vi "GlobalSettings.vi"() -> ()   [LabVIEW 2015]
panel:
  out "Disable Write":bool
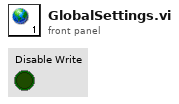
[diagram p1: front panel]
diagram:
